vi "LC Control Get Value.vi"(8 "error in (no error)":errorcluster caption="Error In") -> (0 "error out":errorcluster caption="Error Out")   [LabVIEW 2020]
uses:
  LC Single Control Information.ctl
  LC Mode.ctl
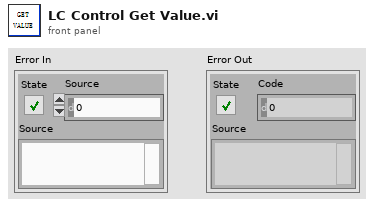
[diagram p1: front panel]
types:
  T1 = typedef "LC Single Control Information.ctl" = cluster{"VI Path":string, "VI Name":string, "Control Name":string, "Property Type":string, "Language":string, "Content":string}
  T2 = typedef "LC Mode.ctl" = enum16{"Init", "NONE", "Read", "Write", "Delete", "Clear", "Save"}
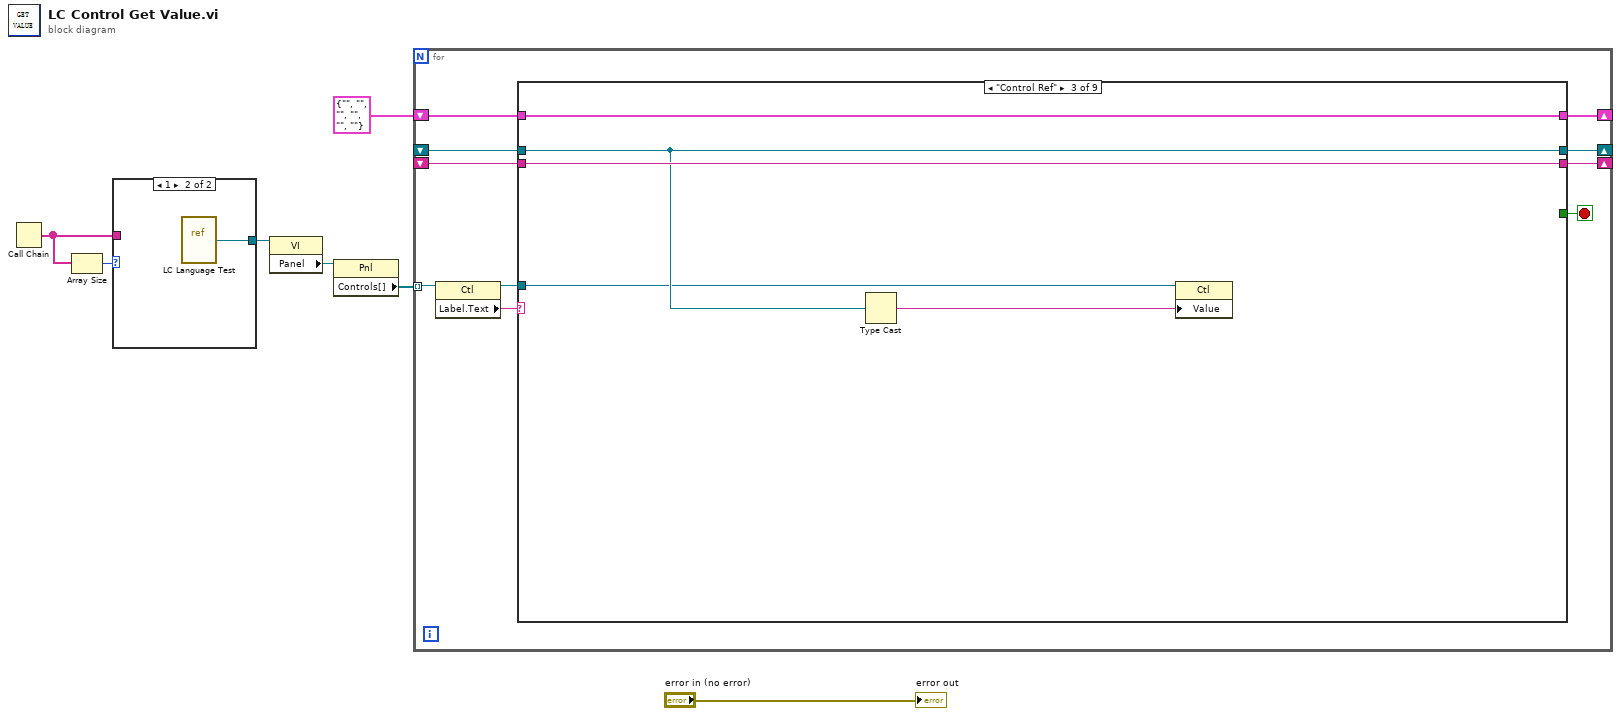
[diagram p0: block diagram]
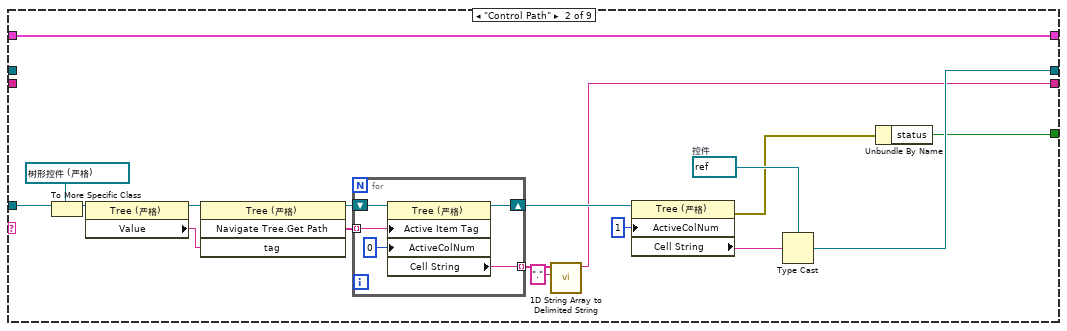
[diagram p3: hidden frame]
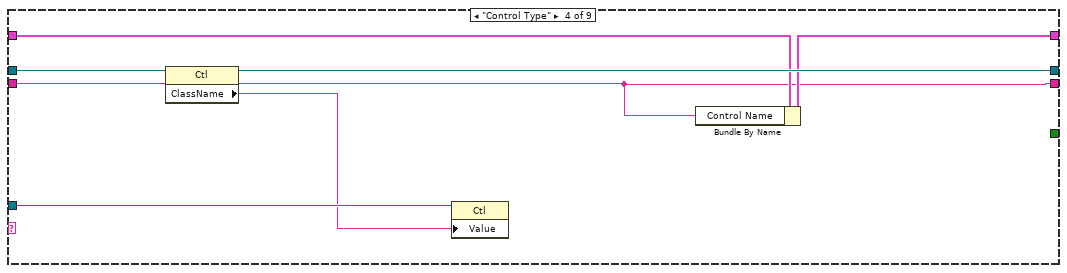
[diagram p4: hidden frame]
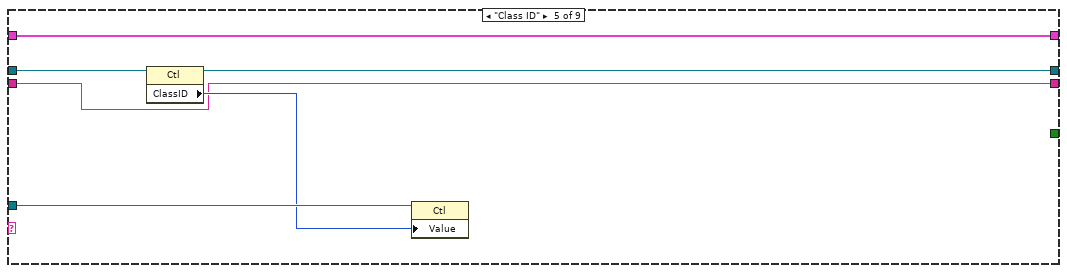
[diagram p5: hidden frame]
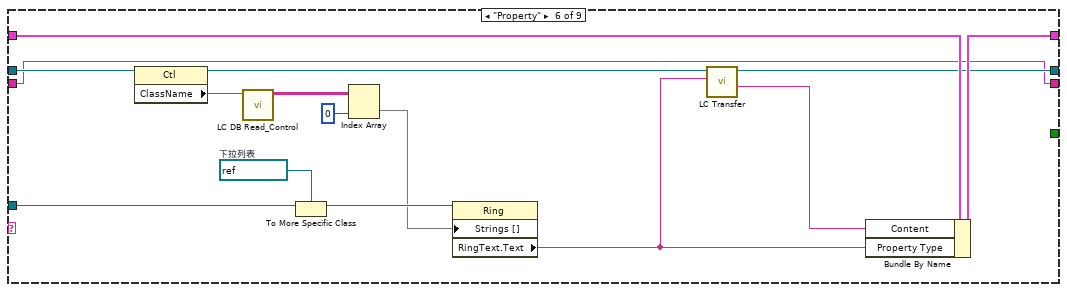
[diagram p6: hidden frame]
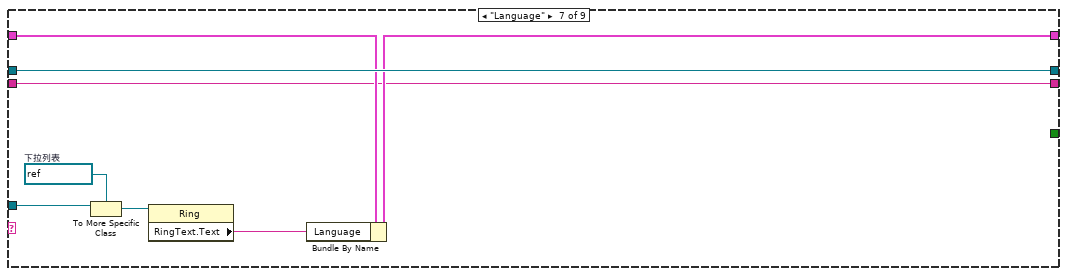
[diagram p7: hidden frame]
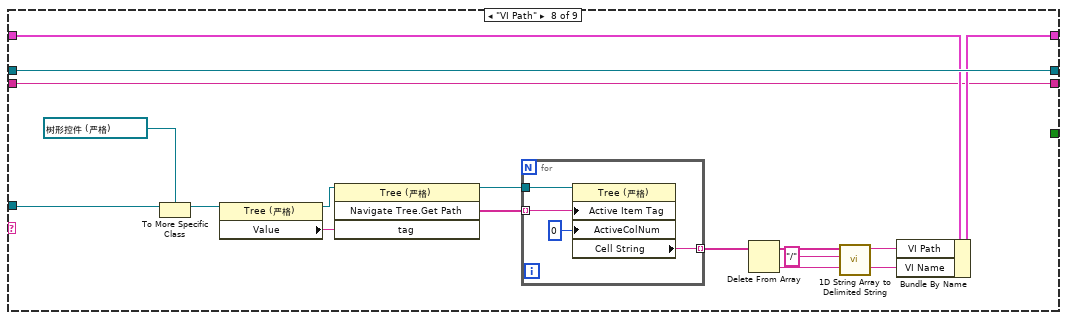
[diagram p8: hidden frame]
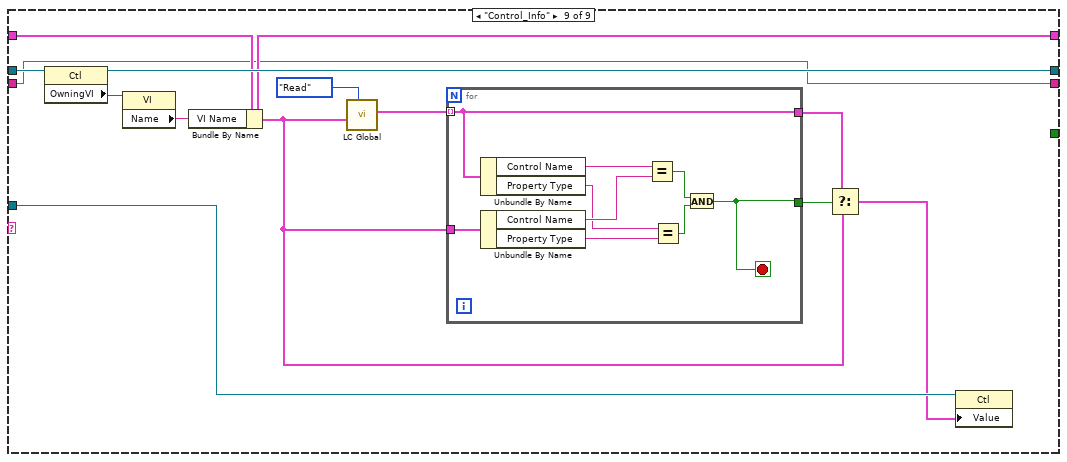
[diagram p9: hidden frame]
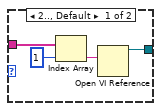
[diagram p10: hidden frame]
diagram:
  n1 = Call Chain() -> (call chain=w4:string[])
  n2 = Array Size(array=w4) -> (size(s)=w5:i32)
  n3 = case shown="1" w5 {
    tunnel: [w9 w12] -> w2
    tunnel: w4 -> [w8 _]
    frame 2.., Default {
      n4 = Index Array(array=w8, index=1 ("索引")) -> (element=w10:string)
      n5 = Open VI Reference(vi path=w10) -> (vi reference=w9:refnum<vi>)  [unwired: 5 in, 1 out]
    }
    frame 1 {
      n6 = vi-ref "LC Language Test.vi"() -> (w12:refnum<vi>)
    }
  }
  n7 = property class="VI"(reference=w2) -> ("Panel"=w3:refnum<vi>)  [unwired: 1 in, 2 out]
  n8 = property class="Pnl"(reference=w3) -> ("Controls[]"=w6:refnum<vi>[])  [unwired: 1 in, 2 out]
  n9 = for {
    tunnel: w6 -> [w22] mode=indexing
    shift-right: [w18] -> _
    shift-left: _ -> [w19]
    shift-right: [w15] -> _
    shift-left: T1 {"VI Path"="", "VI Name"="", "Control Name"="", "Property Type"="", "Language"="", "Content"=""} ("Write") -> [w16]
    shift-right: [w14] -> _
    shift-left: _ -> [w13]
    stop <- w17 stop-if-true
    n10 = property class="Ctl"(reference=w22) -> (reference out=w20:refnum<vi>, "Label.Text"=w21:string)  [unwired: 1 in, 1 out]
    n11 = case shown="\"Control Ref\"" w21 {
      tunnel: w20 -> [_ w41 w50 w58 w64 w76 w88 w96 w115]
      tunnel: w19 -> [w25 _ w51 w60 w66 w81 w89 w105 w121]
      tunnel: [w25 w40 w51 w59 w65 w70 w89 w105 w120] -> w18
      tunnel: [_ w38 _ _ _ _ _ _ _] -> w17
      tunnel: w16 -> [w24 w37 w53 w56 w62 w73 w85 w95 w118]
      tunnel: [w24 w37 w53 w55 w62 w72 w84 w94 w111] -> w15
      tunnel: [w23 w26 w52 w54 w61 w67 w82 w90 w110] -> w14
      tunnel: w13 -> [w23 _ w52 w54 w61 w67 w82 w90 w110]
      frame "eee", Default {
      }
      frame "Control Path" {
        w42 = refnum<vi> refnum  # 控件
        n12 = To More Specific Class(target class=refnum<vi> refnum ("引用输出"), reference=w41) -> (specific class reference=w30:refnum<vi>)  [unwired: 1 in, 1 out]
        n13 = property class="Tree (严格)"(reference=w30) -> (reference out=w33:refnum<vi>, "Value"=w32:string)  [unwired: 1 in, 1 out]
        n14 = invoke class="Tree (严格)" method="Navigate Tree.Get Path"(reference=w33, "tag"=w32) -> (reference out=w35:refnum<vi>, "Navigate Tree:Get Path"=w34:string[])  [unwired: 2 in, 2 out]
        n15 = for {
          tunnel: w34 -> [w47] mode=indexing
          tunnel: [w46] -> w28 mode=indexing
          shift-right: [w44] -> w29
          shift-left: w35 -> [w45]
          n16 = property class="Tree (严格)"(reference=w45, "Active Item Tag"=w47, "ActiveColNum"=0 ("活动单元格:活动列数")) -> (reference out=w44:refnum<vi>, "Cell String"=w46:string)  [unwired: 1 in, 1 out]
        }
        n17 = call <vilib>:"1D String Array to Delimited String.vi"("delimiter"=".", "string array"=w28) -> ("delimited string"=w26:string)  [unwired: 9 in]
        n18 = property class="Tree (严格)"(reference=w29, "ActiveColNum"=1 ("活动单元格:活动列数")) -> (error out=w39:errorcluster, "Cell String"=w43:string)  [unwired: 1 in, 1 out]
        n19 = Type Cast(type=w42, x=w43) -> (*(type *) &x=w40:refnum<vi>)
        n20 = Unbundle By Name(w39) -> ("status"=w38:bool)
      }
      frame "Control Ref" {
        n21 = Type Cast(x=w51) -> (*(type *) &x=w49:string)  [unwired: 1 in]
        n22 = property class="Ctl"(reference=w50, "Value"=w49) -> ()  [unwired: 1 in, 2 out]
      }
      frame "Control Type" {
        n23 = property class="Ctl"(reference=w60) -> (reference out=w59:refnum<vi>, "ClassName"=w57:string)  [unwired: 1 in, 1 out]
        n24 = property class="Ctl"(reference=w58, "Value"=w57) -> ()  [unwired: 1 in, 2 out]
        n25 = Bundle By Name(cluster=w56, "Control Name"=w54) -> (w55:T1)
      }
      frame "Class ID" {
        n26 = property class="Ctl"(reference=w66) -> (reference out=w65:refnum<vi>, "ClassID"=w63:u32)  [unwired: 1 in, 1 out]
        n27 = property class="Ctl"(reference=w64, "Value"=w63) -> ()  [unwired: 1 in, 2 out]
      }
      frame "Property" {
        w77 = refnum<vi> refnum  # 下拉列表
        n28 = property class="Ctl"(reference=w81) -> (reference out=w71:refnum<vi>, "ClassName"=w78:string)  [unwired: 1 in, 1 out]
        n29 = call "LC DB Read_Control.vi"("Table Name"=w78) -> ("Data"=w80:string[][])  [unwired: 9 in, 1 out]
        n30 = To More Specific Class(target class=w77, reference=w76) -> (specific class reference=w75:refnum<vi>)  [unwired: 1 in, 1 out]
        n31 = Index Array(array=w80, index (col)=0 ("禁用的索引 (列)")) -> (element=w74:string[])  [unwired: 1 in]
        n32 = property class="Ring"(reference=w75, "Strings []"=w74) -> ("RingText.Text"=w68:string)  [unwired: 1 in, 2 out]
        n33 = call "LC Transfer.vi"("Property"=w68, "Ctl Ref In"=w71) -> ("Value Out"=w69:string, "Ctl Ref Out"=w70:refnum<vi>)  [unwired: 7 in, 1 out]
        n34 = Bundle By Name(cluster=w73, "Content"=w69, "Property Type"=w68) -> (w72:T1)
      }
      frame "Language" {
        w87 = refnum<vi> refnum  # 下拉列表
        n35 = To More Specific Class(target class=w87, reference=w88) -> (specific class reference=w86:refnum<vi>)  [unwired: 1 in, 1 out]
        n36 = property class="Ring"(reference=w86) -> ("RingText.Text"=w83:string)  [unwired: 1 in, 2 out]
        n37 = Bundle By Name(cluster=w85, "Language"=w83) -> (w84:T1)
      }
      frame "VI Path" {
        n38 = To More Specific Class(target class=refnum<vi> refnum ("引用输出"), reference=w96) -> (specific class reference=w103:refnum<vi>)  [unwired: 1 in, 1 out]
        n39 = property class="Tree (严格)"(reference=w103) -> (reference out=w99:refnum<vi>, "Value"=w98:string)  [unwired: 1 in, 1 out]
        n40 = invoke class="Tree (严格)" method="Navigate Tree.Get Path"(reference=w99, "tag"=w98) -> (reference out=w102:refnum<vi>, "Navigate Tree:Get Path"=w100:string[])  [unwired: 2 in, 2 out]
        n41 = for {
          tunnel: w100 -> [w108] mode=indexing
          tunnel: [w107] -> w101 mode=indexing
          tunnel: w102 -> [w106]
          n42 = property class="Tree (严格)"(reference=w106, "Active Item Tag"=w108, "ActiveColNum"=0 ("活动单元格:活动列数")) -> ("Cell String"=w107:string)  [unwired: 1 in, 2 out]
        }
        n43 = Delete From Array(array=w101) -> (deleted portion=w104:string, array with subset deleted=w93:string[])  [unwired: 2 in]
        n44 = call <vilib>:"1D String Array to Delimited String.vi"("delimiter"="/", "string array"=w93) -> ("delimited string"=w91:string)  [unwired: 9 in]
        n45 = Bundle By Name(cluster=w95, "VI Path"=w91, "VI Name"=w104) -> (w94:T1)
      }
      frame "Control_Info" {
        n46 = property class="Ctl"(reference=w121) -> (reference out=w120:refnum<vi>, "OwningVI"=w119:refnum<vi>)  [unwired: 1 in, 1 out]
        n47 = property class="VI"(reference=w119) -> ("Name"=w117:string)  [unwired: 1 in, 2 out]
        n48 = Bundle By Name(cluster=w118, "VI Name"=w117) -> (w111:T1)
        n49 = call "LC Global.vi"("Mode"=LC_Mode."Read", "Write"=w111) -> ("Read"=w116:T1[])  [unwired: 7 in, 2 out]
        n50 = for {
          tunnel: w116 -> [w127] mode=indexing
          tunnel: w111 -> [w125]
          tunnel: [w127] -> w113
          tunnel: [w126] -> w114
          stop <- w126 stop-if-true
          n51 = Unbundle By Name(w127) -> ("Control Name"=w131:string, "Property Type"=w124:string)
          n52 = Unbundle By Name(w125) -> ("Control Name"=w130:string, "Property Type"=w123:string)
          n53 = Equal?(x=w131, y=w130) -> (x = y?=w129:bool)
          n54 = Equal?(x=w124, y=w123) -> (x = y?=w128:bool)
          n55 = And(x=w129, y=w128) -> (x .and. y?=w126:bool)
        }
        n56 = Select(t=w113, s=w114, f=w111) -> (s? t:f=w112:T1)
        n57 = property class="Ctl"(reference=w115, "Value"=w112) -> ()  [unwired: 1 in, 2 out]
      }
    }
  }
  "error out" <- "error in (no error)"
